vi "Differentiate.vi"(8 "error in (no error)":errorcluster, 9 "Baratron 2":dbl, 10 "Baratron 1":dbl, 11 "cRIO Vacuum in":refnum<class "cRIO Vacuum.lvclass">) -> (0 "error out":errorcluster, 1 "d/dt 2":dbl, 2 "d/dt 1":dbl, 3 "cRIO Vacuum out":refnum<class "cRIO Vacuum.lvclass">)   [LabVIEW 2015, in "cRIO-Carbondioxide.lvlib" / "CO2-Actor.lvlib" / "cRIO Vacuum.lvclass"]
uses:
  cRIO Vacuum.lvclass
  <vilib>/ptbypt/NI_PtbyPt.lvlib
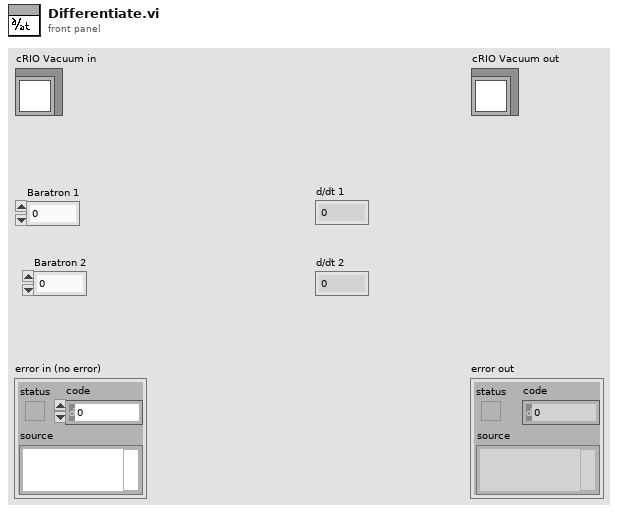
[diagram p1: front panel]
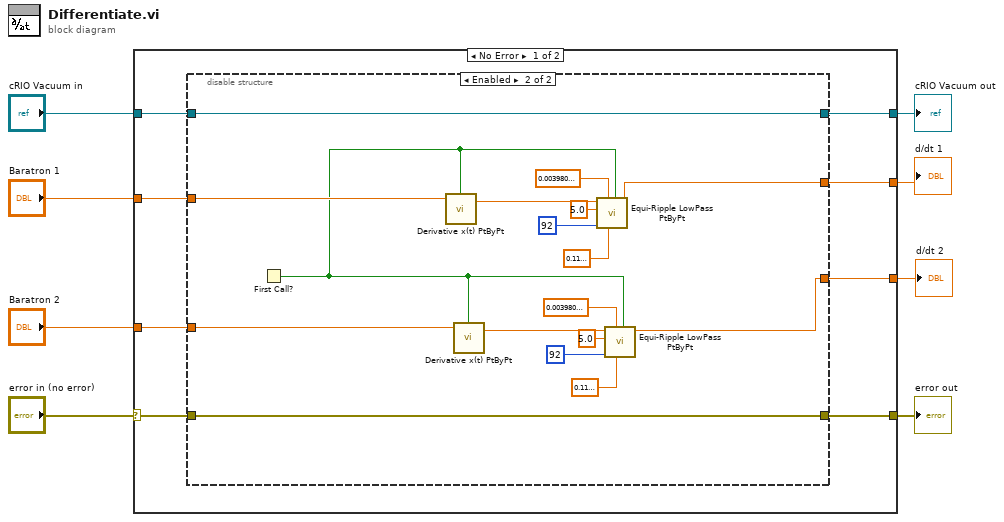
[diagram p0: block diagram]
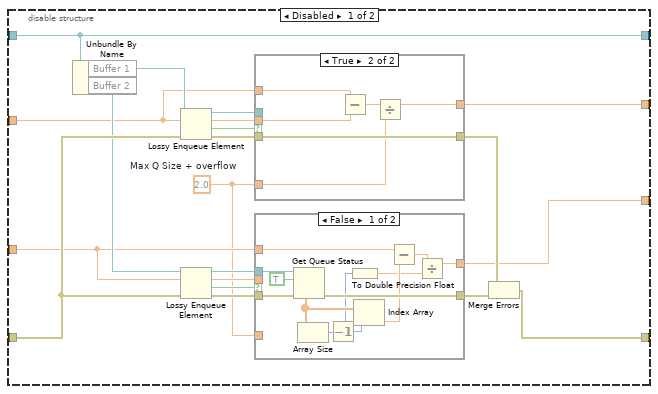
[diagram p2: hidden frame]
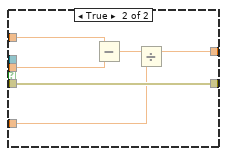
[diagram p3: hidden frame]
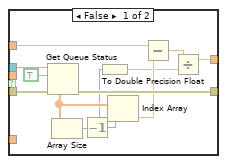
[diagram p4: hidden frame]
diagram:
  n1 = case shown="No Error" "error in (no error)" {
    selector: "error in (no error)" -> [w15 w90]
    tunnel: [w12 w90] -> w7
    tunnel: [w9 w91] -> w5
    tunnel: "cRIO Vacuum in" -> [w16 w91]
    tunnel: "Baratron 1" -> [w14 _]
    tunnel: "Baratron 2" -> [w13 _]
    tunnel: [w10 _] -> w2
    tunnel: [w11 _] -> w1
    frame No Error {
      n2 = disable-structure shown="Enabled" {
        disable-tunnel: w16 -> [w17 w89]
        disable-tunnel: w15 -> [w35 w88]
        disable-tunnel: w14 -> [w30 w75]
        disable-tunnel: w13 -> [w28 w87]
        disable-tunnel: [w21 w88] -> w12
        disable-tunnel: [w19 w74] -> w11
        disable-tunnel: [w18 w81] -> w10
        disable-tunnel: [w17 w89] -> w9
        frame Disabled {
          w20 = 2.0  # Max Q Size + overflow
          n3 = Unbundle By Name(w17) -> ("Buffer 1"=w36:refnum<queue>, "Buffer 2"=w34:refnum<queue>)
          n4 = Lossy Enqueue Element(queue=w36, element=w30, error in (no error)=w35) -> (queue out=w31:refnum<queue>, overflow element=w29:dbl, overflow?=w32:bool, error out=w33:errorcluster)
          n5 = Lossy Enqueue Element(queue=w34, element=w28, error in (no error)=w35) -> (queue out=w25:refnum<queue>, overflow element=w24:dbl, overflow?=w26:bool, error out=w27:errorcluster)
          n6 = case shown="True" w32 {
            tunnel: w33 -> [w66 w69]
            tunnel: w31 -> [w65 _]
            tunnel: w30 -> [w59 w72]
            tunnel: w29 -> [_ w71]
            tunnel: [w58 w68] -> w19
            tunnel: [w61 w69] -> w22
            tunnel: w20 -> [_ w67]
            frame False {
              n7 = Get Queue Status(queue=w65, return elements? (F)=TRUE, error in (no error)=w66) -> (error out=w61:errorcluster, elements=w63:dbl[])  [unwired: 6 out]
              n8 = Array Size(array=w63) -> (size(s)=w57:i32)
              n9 = Decrement(x=w57) -> (x-1=w62:i32)
              n10 = To Double Precision Float(number=w57) -> (double precision float=w55:dbl)
              n11 = Index Array(array=w63, index=w62) -> (element=w60:dbl)
              n12 = Subtract(x=w59, y=w60) -> (x-y=w56:dbl)
              n13 = Divide(x=w56, y=w55) -> (x/y=w58:dbl)
            }
            frame True {
              n14 = Subtract(x=w72, y=w71) -> (x-y=w70:dbl)
              n15 = Divide(x=w70, y=w67) -> (x/y=w68:dbl)
            }
          }
          n16 = case shown="False" w26 {
            tunnel: w27 -> [w48 w51]
            tunnel: w25 -> [w47 _]
            tunnel: w28 -> [w41 w54]
            tunnel: w24 -> [_ w53]
            tunnel: [w40 w50] -> w18
            tunnel: [w43 w51] -> w23
            tunnel: w20 -> [_ w49]
            frame False {
              n17 = Get Queue Status(queue=w47, return elements? (F)=TRUE, error in (no error)=w48) -> (error out=w43:errorcluster, elements=w45:dbl[])  [unwired: 6 out]
              n18 = Array Size(array=w45) -> (size(s)=w39:i32)
              n19 = Decrement(x=w39) -> (x-1=w44:i32)
              n20 = To Double Precision Float(number=w39) -> (double precision float=w38:dbl)
              n21 = Index Array(array=w45, index=w44) -> (element=w42:dbl)
              n22 = Subtract(x=w41, y=w42) -> (x-y=w37:dbl)
              n23 = Divide(x=w37, y=w38) -> (x/y=w40:dbl)
            }
            frame True {
              n24 = Subtract(x=w54, y=w53) -> (x-y=w52:dbl)
              n25 = Divide(x=w52, y=w49) -> (x/y=w50:dbl)
            }
          }
          n26 = Merge Errors(w22, w23) -> (w21:errorcluster)
        }
        frame Enabled {
          n27 = First Call?() -> (First Call?: T/F=w73:bool)
          n28 = call <vilib>:"Derivative x(t) PtByPt.vi"("initialize"=w73, "x"=w75) -> ("dx/dt"=w76:dbl)  [unwired: 2 in, 1 out]
          n29 = call <vilib>:"Derivative x(t) PtByPt.vi"("initialize"=w73, "x"=w87) -> ("dx/dt"=w86:dbl)  [unwired: 2 in, 1 out]
          n30 = call <vilib>:"Equi-Ripple LowPass PtByPt.vi"("initialize"=w73, "stop freq"=0.1199999999999999 ("stop freq 2"), "pass freq"=0.003980000000000005 ("pass freq 2"), "# of taps"=92 ("# of taps 2"), "sampling freq: fs"=5.0, "x"=w76) -> ("Filtered x"=w74:dbl)  [unwired: 3 in, 1 out]
          n31 = call <vilib>:"Equi-Ripple LowPass PtByPt.vi"("initialize"=w73, "stop freq"=0.1199999999999999 ("stop freq 2"), "pass freq"=0.003980000000000005 ("pass freq 2"), "# of taps"=92 ("# of taps 2"), "sampling freq: fs"=5.0, "x"=w86) -> ("Filtered x"=w81:dbl)  [unwired: 3 in, 1 out]
        }
      }
    }
    frame Error {
    }
  }
  "error out" <- w7
  "cRIO Vacuum out" <- w5
  "d/dt 2" <- w2
  "d/dt 1" <- w1
